vi "generate signal.vi"(10 "Phase":dbl) -> (2 "Waveform":waveform(dbl))   [LabVIEW 2020]
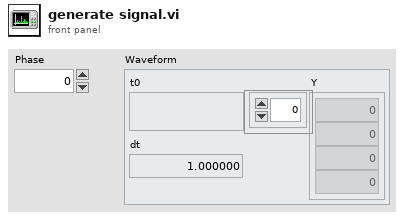
[diagram p1: front panel]
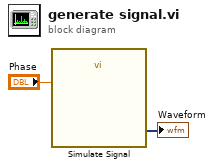
[diagram p0: block diagram]
diagram:
  n1 = call "Simulate Signal"("Phase"="Phase") -> ("Sine"=→"Waveform":dynamicdata)  [unwired: 13 in, 1 out]
